vi "Get RFPM Device Temperature.vi"(0 "IVISwitch Handle in":refnum<k15>, 11 "error in":errorcluster) -> (4 "IVISwitch Handle out":refnum<k15>, 6 "Device Temperature":dbl, 15 "error out":errorcluster)   [LabVIEW 2023, in "RFFixtureCharact.RFPM.lvlib" / "RF Subsystem Session Provider.lvclass"]
uses:
  RF Subsystem Session Provider.lvclass
  niRFPMSwitch_64.dll
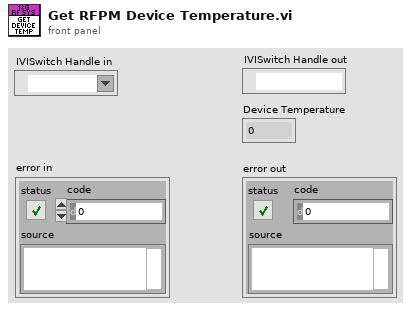
[diagram p1: front panel]
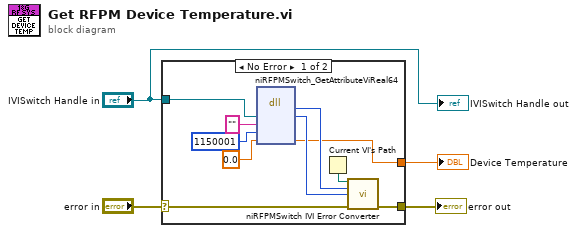
[diagram p0: block diagram]
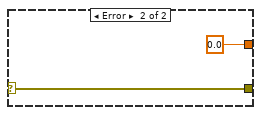
[diagram p2: hidden frame]
diagram:
  n1 = case shown="No Error" "error in" {
    selector: "error in" -> [w7 w16]
    tunnel: "IVISwitch Handle in" -> [w8 _]
    tunnel: [w6 w16] -> w4
    tunnel: [w5 0.0 ("Device Temperature")] -> w3
    frame No Error {
      n2 = dll-call lib="niRFPMSwitch**.*" fn="niRFPMSwitch_GetAttributeViReal64" ("ni5530SParameterLibrary.dll:ni5530SParameterLibrary_ConfigureResources")("instrument handle"=w8, "ChannelName"="", "Attribute"=u32 1150001, "Value"=0.0) -> ("Status"=w13:i32, "instrument handle"=w14:u32, "Value"=w5:dbl)  [unwired: 3 in, 4 out]
      n3 = Current VI's Path() -> (path=w12:path)
      n4 = call <instrlib>:"niRFPMSwitch IVI Error Converter.vi"("path to vi"=w12, "ivi error code"=w13, "instrument handle"=w14, "error in"=w7) -> ("error out"=w6:errorcluster)  [unwired: 11 in]
    }
    frame Error {
    }
  }
  "error out" <- w4
  "Device Temperature" <- w3
  "IVISwitch Handle out" <- "IVISwitch Handle in"
